vi "Read File.vi"(8 "error in (no error)":errorcluster) -> (0 "error out":errorcluster, 3 "Account Details":T1(array[cluster]))   [LabVIEW 2019, in "SubVI.lvlib"]
uses:
  <vilib>/Utility/file.llb/Read Delimited Spreadsheet (string).vi
  SubVIs/SubVI.lvlib
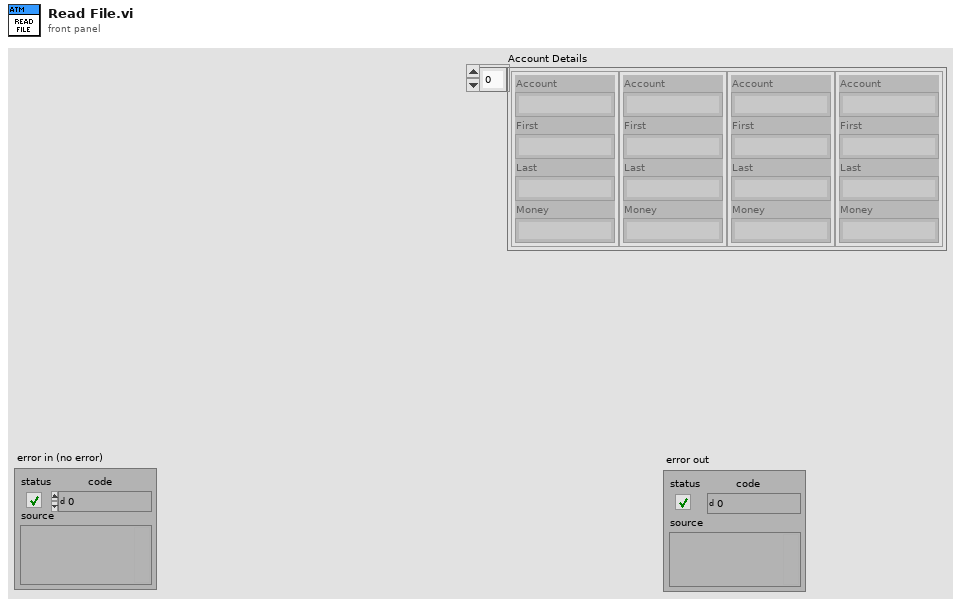
[diagram p1: front panel]
types:
  T1 = cluster{"Account":string, "First":string, "Last":string, "Money":string}[]
  T2 = cluster{"Account":string, "First":string, "Last":string, "Money":string}
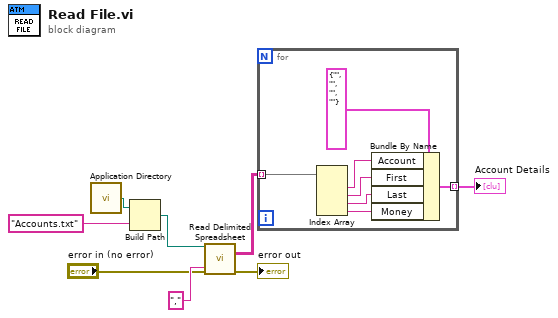
[diagram p0: block diagram]
diagram:
  n1 = call <vilib>:"Application Directory.vi"() -> ("Application Directory"=w8:path)
  n2 = Build Path(base path=w8, name or relative path="Accounts.txt") -> (appended path=w6:path)
  n3 = call-poly <vilib>:"Read Delimited Spreadsheet.vi"("file path (dialog if empty)"=w6, "error in (no error)"="error in (no error)", "delimiter (\\t)"="," ("delimiter (\\t)")) -> ("all rows"=w4:string[][], "error out"=→"error out":errorcluster)  [unwired: 7 in, 4 out]
  n4 = for {
    tunnel: w4 -> [w15] mode=indexing
    tunnel: [w10] -> w3 mode=indexing
    n5 = Index Array(array=w15) -> (element #1=w14:string, element #2=w13:string, element #3=w12:string, element #4=w11:string)  [unwired: 4 in]
    n6 = Bundle By Name(cluster=T2 {"Account"="", "First"="", "Last"="", "Money"=""}, "Account"=w14, "First"=w13, "Last"=w12, "Money"=w11) -> (w10:T2)
  }
  "Account Details" <- w3
